vi "IPC-Initialize.vi"() -> (0 "error IO":errorcluster)   [LabVIEW 2014]
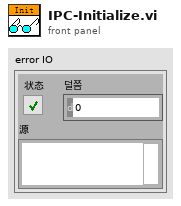
[diagram p1: front panel]
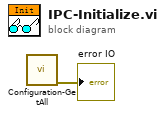
[diagram p0: block diagram]
diagram:
  n1 = call "Configuration-GetAll.vi"() -> ("error IO"=→"error IO":errorcluster)  [unwired: 10 in]
